vi "shotnoise.vi"() -> ()   [LabVIEW 2013]
panel:
  out "count":i64
  out "sn":dbl[](array[numeric])=[1.0, 1.0]
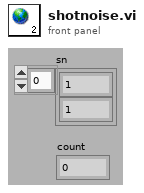
[diagram p1: front panel]
diagram:
